vi "initializeStyle.vi"(8 "error in (no error)":errorcluster, 10 "Style":refnum<class "Style.lvclass">, 11 "xwpfRun.Normal in":refnum<class "xwpfRun.Normal.lvclass">) -> (0 "error out":errorcluster, 3 "xwpfRun.Normal out":refnum<class "xwpfRun.Normal.lvclass">)   [LabVIEW 2017, in "Word_Specific.lvlib" / "xwpfRun.Normal.lvclass"]
uses:
  xwpfRun.Normal.lvclass
  Styles/Style/Style.lvclass
  xwpfRun/xwpfRun.lvclass
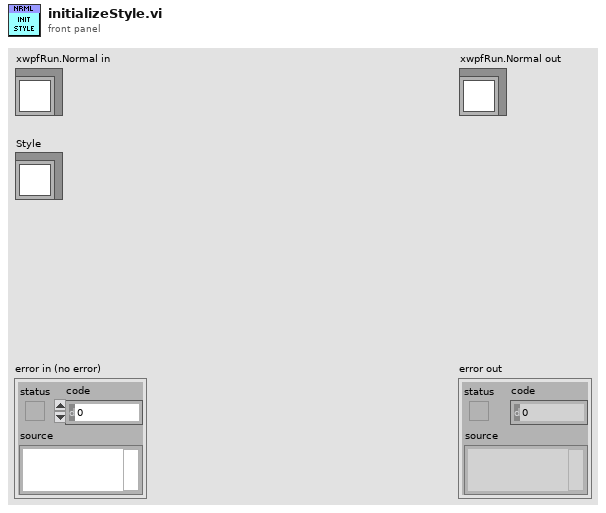
[diagram p1: front panel]
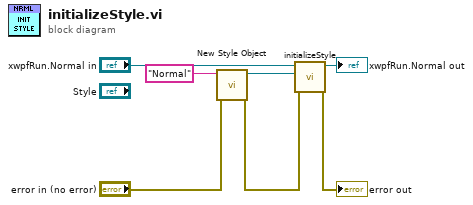
[diagram p0: block diagram]
diagram:
  n1 = call "New Style Object.vi"("error in (no error)"="error in (no error)", "Style Name"="Normal") -> ("error out"=w2:errorcluster, "Style out"=w4:refnum<class "Style.lvclass">)  [unwired: 8 in]
  n2 = call-parent "initializeStyle.vi"("error in (no error)"=w2, "Style"=w4, "xwpfRun in"="xwpfRun.Normal in") -> ("error out"=→"error out":errorcluster, "xwpfRun out"=→"xwpfRun.Normal out":refnum<class "xwpfRun.Normal.lvclass">)  [unwired: 7 in]
